vi "Launch SmallView.vi"(8 "error in (no error)":errorcluster, 11 "Sensor in":refnum<class "Sensor.lvclass">) -> (0 "error out":errorcluster, 3 "Sensor out":refnum<class "Sensor.lvclass">)   [LabVIEW 2012, in "Sensor Definition.lvlib" / "Sensor.lvclass"]
uses:
  Sensor.lvclass
  <vilib>/ActorFramework/Actor/Actor.lvclass
  DemoMain Messages/Display in Grid Msg/Display in Grid Msg.lvclass
  HostType.ctl
  Sensor Definition.lvlib
  SensorViewSmall.lvclass
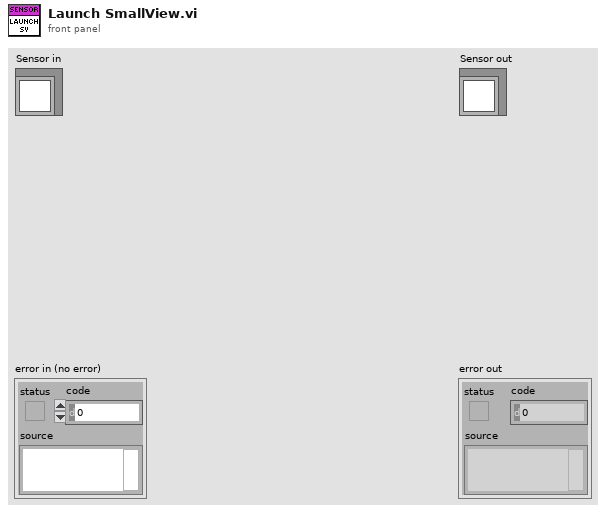
[diagram p1: front panel]
types:
  T1 = typedef "Sensor Definition.lvlib/HostType.ctl" = enum16{"Standalone", "Grid", "MainPane"}
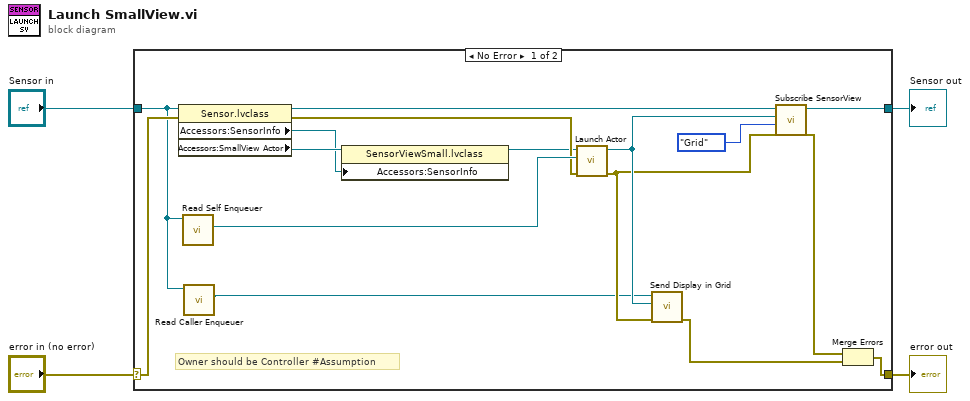
[diagram p0: block diagram]
diagram:
  n1 = case shown="No Error" "error in (no error)" {
    selector: "error in (no error)" -> [w18 w22]
    tunnel: [w14 w22] -> w3
    tunnel: [w9 w21] -> w1
    tunnel: "Sensor in" -> [w6 w21]
    frame No Error {
      # "Owner should be Controller #Assumption"
      n2 = property class="Sensor.lvclass"(reference=w6, error in=w18) -> (reference out=w16:refnum<class "Sensor.lvclass">, error out=w17:errorcluster, "Accessors:SensorInfo"=w7:refnum<class "SensorInfo.lvclass">, "Accessors:SmallView Actor"=w20:refnum<class "SensorViewSmall.lvclass">)
      n3 = call <vilib>:"Read Self Enqueuer.vi"("Actor"=w6) -> ("Self Enqueuer"=w19:refnum<class "Message Enqueuer.lvclass">)  [unwired: 10 in]
      n4 = call <vilib>:"Read Caller Enqueuer.vi"("Actor"=w6) -> ("Caller Enqueuer"=w5:refnum<class "Message Enqueuer.lvclass">)  [unwired: 10 in]
      n5 = property class="SensorViewSmall.lvclass"(reference=w20, "Accessors:SensorInfo"=w7) -> (reference out=w8:refnum<class "SensorViewSmall.lvclass">)  [unwired: 1 in, 1 out]
      n6 = call <vilib>:"Launch Actor.vi"("error in (no error)"=w17, "Actor-to-Caller Enqueuer"=w19, "Actor"=w8) -> ("error out"=w12:errorcluster, "Caller-To-Actor Enqueuer"=w13:refnum<class "Message Enqueuer.lvclass">)  [unwired: 7 in]
      n7 = call "Send Display in Grid.vi"("error in (no error)"=w12, "ViewableActor"=w13, "Message Enqueuer"=w5) -> ("error out"=w11:errorcluster)  [unwired: 7 in, 1 out]
      n8 = call "Subscribe SensorView.vi"("error in (no error)"=w12, "HostType"=HostType."Grid", "SensorView Enqueuer"=w13, "Sensor in"=w16) -> ("error out"=w15:errorcluster, "Sensor out"=w9:refnum<class "Sensor.lvclass">)  [unwired: 6 in]
      n9 = Merge Errors(w15, w11) -> (w14:errorcluster)
    }
    frame Error {
    }
  }
  "error out" <- w3
  "Sensor out" <- w1
